vi "is valid path.vi"(1 "Path":path) -> (0 "Is valid path?":bool)   [LabVIEW 2022 SP3]
doc: "This VI returns True if and only if the input path is valid.\n\nA valid path is a path that:\n1. Is not \"Empty path\"\nAND\n2. Is not \"Not a Path\""
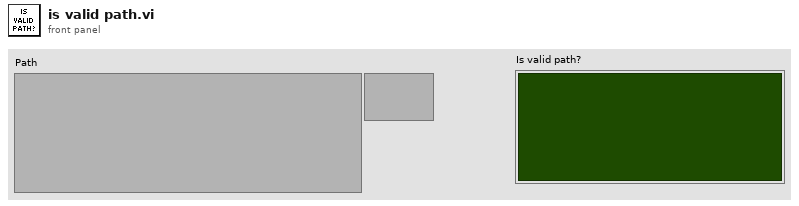
[diagram p1: front panel]
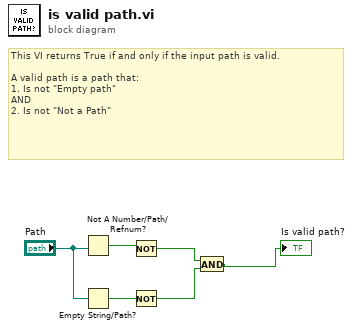
[diagram p0: block diagram]
diagram:
  # "This VI returns True if and only if the input path is valid.\n\nA valid path is a path that:\n1. Is not \"Empty path\"\nAND\n2. Is not \"Not a Path\""
  n1 = Not A Number/Path/Refnum?(number/path/refnum="Path") -> (NaN/Path/Refnum?=w5:bool)
  n2 = Empty String/Path?(string/path="Path") -> (empty?=w4:bool)
  n3 = Not(x=w5) -> (.not. x?=w3:bool)
  n4 = Not(x=w4) -> (.not. x?=w2:bool)
  n5 = And(x=w3, y=w2) -> (x .and. y?=→"Is valid path?":bool)
